vi "SP Get All Plot References.vi"(1 "Plots Tab Control":refnum<vi>) -> (0 "Plot References":refnum<vi>[](array[refnum]))   [LabVIEW 2011]
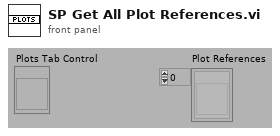
[diagram p1: front panel]
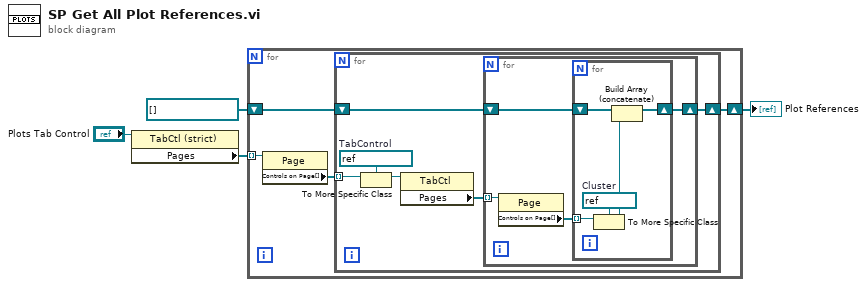
[diagram p0: block diagram]
diagram:
  n1 = property class="TabCtl (strict)"(reference="Plots Tab Control") -> ("Pages"=w3:refnum<vi>[])  [unwired: 1 in, 2 out]
  n2 = for {
    tunnel: w3 -> [w6] mode=indexing
    shift-right: [w7] -> w2
    shift-left: refnum<vi>[] [] -> [w8]
    n3 = property class="Page"(reference=w6) -> ("Controls on Page[]"=w5:refnum<vi>[])  [unwired: 1 in, 2 out]
    n4 = for {
      tunnel: w5 -> [w12] mode=indexing
      shift-right: [w13] -> w7
      shift-left: w8 -> [w14]
      w11 = refnum<vi> refnum  # TabControl
      n5 = To More Specific Class(target class=w11, reference=w12) -> (specific class reference=w10:refnum<vi>)  [unwired: 1 in, 1 out]
      n6 = property class="TabCtl"(reference=w10) -> ("Pages"=w9:refnum<vi>[])  [unwired: 1 in, 2 out]
      n7 = for {
        tunnel: w9 -> [w16] mode=indexing
        shift-right: [w17] -> w13
        shift-left: w14 -> [w18]
        n8 = property class="Page"(reference=w16) -> ("Controls on Page[]"=w15:refnum<vi>[])  [unwired: 1 in, 2 out]
        n9 = for {
          tunnel: w15 -> [w22] mode=indexing
          shift-right: [w19] -> w17
          shift-left: w18 -> [w21]
          w23 = refnum<vi> refnum  # Cluster
          n10 = To More Specific Class(target class=w23, reference=w22) -> (specific class reference=w20:refnum<vi>)  [unwired: 1 in, 1 out]
          n11 = Build Array (concatenate)(w21, w20) -> (w19:refnum<vi>[])
        }
      }
    }
  }
  "Plot References" <- w2
